vi "Load Device Image.vi"(8 "Error In":errorcluster, 10 "Device Type":u16(ring) items=["chipKIT Uno32", "chipKIT uC32", "chipKIT Max32", "chipKIT DP32"], 11 "Device Family":u16(ring) items=["National Instruments", "Digilent", "Arduino"]) -> (0 "Error Out":errorcluster, 3 "Device Image":picture)   [LabVIEW 2011, in "LVH-LINX.lvlib"]
doc: "Load LINX Device Image"
uses:
  LVH-LINX.lvlib
  <vilib>/LabVIEW Hacker/LVH-Toolbox/Common/LVH-Common.lvlib
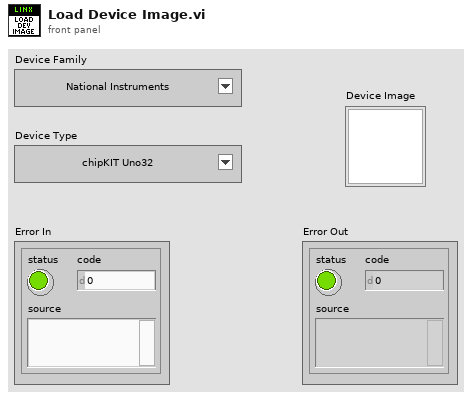
[diagram p1: front panel]
types:
  T1 = typedef "imagedata.ctl" = cluster{"image type":i32, "image depth":i32, "image":u8[], "mask":u8[], "colors":u32[], "Rectangle":cluster{"left":i16, "top":i16, "right":i16, "bottom":i16}}
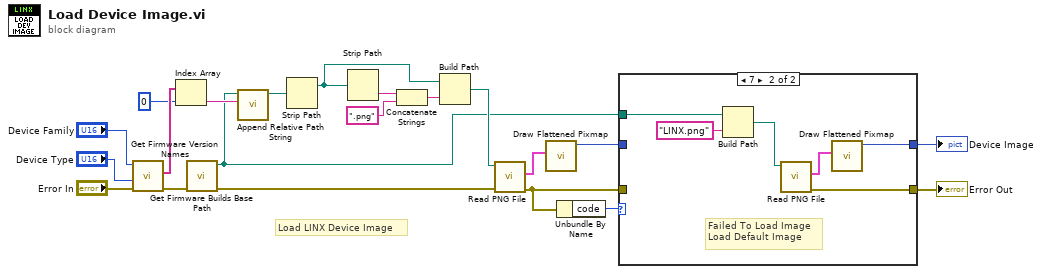
[diagram p0: block diagram]
diagram:
  # "Load LINX Device Image"
  n1 = call "Get Firmware Version Names.vi"("Error In"="Error In", "Device ID"="Device Type", "Device Family"="Device Family") -> ("Error Out"=w20:errorcluster, "Firmware Version Relative Path"=w21:string[])  [unwired: 6 in, 1 out]
  n2 = Index Array(array=w21, index=0) -> (element=w19:string)
  n3 = call "Get Firmware Builds Base Path.vi"("Error In"=w20) -> ("Error Out"=w8:errorcluster, "Firmware Builds Base Path"=w1:path)  [unwired: 9 in]
  n4 = call <vilib>:"Append Relative Path String.vi"("Relative Path"=w19, "Base Path"=w1) -> ("Absolute Path"=w14:path)  [unwired: 9 in]
  n5 = Strip Path(path=w14) -> (stripped path=w11:path)  [unwired: 1 out]
  n6 = Strip Path(path=w11) -> (name=w13:string)  [unwired: 1 out]
  n7 = Concatenate Strings(w13, ".png" ("string")) -> (w10:string)
  n8 = Build Path(base path=w11, name or relative path=w10) -> (appended path=w9:path)
  n9 = call <vilib>:"Read PNG File.vi"("error in (no error)"=w8, "path to PNG file"=w9) -> ("error out"=w5:errorcluster, "image data"=w7:T1)  [unwired: 7 in, 1 out]
  n10 = call <vilib>:"Draw Flattened Pixmap.vi"("image data"=w7) -> ("new picture"=w2:picture)  [unwired: 8 in]
  n11 = Unbundle By Name(w5) -> ("code"=w6:i32)
  n12 = case shown="7" w6 {
    tunnel: w5 -> [w22 _]
    tunnel: [w22 w25] -> w4
    tunnel: [w23 w26] -> w3
    tunnel: w2 -> [w23 _]
    tunnel: w1 -> [_ w29]
    frame 0, Default {
    }
    frame 7 {
      # "Failed To Load Image\nLoad Default Image"
      n13 = Build Path(base path=w29, name or relative path="LINX.png") -> (appended path=w24:path)
      n14 = call <vilib>:"Read PNG File.vi"("path to PNG file"=w24) -> ("error out"=w25:errorcluster, "image data"=w28:T1)  [unwired: 8 in, 1 out]
      n15 = call <vilib>:"Draw Flattened Pixmap.vi"("image data"=w28) -> ("new picture"=w26:picture)  [unwired: 8 in]
    }
  }
  "Error Out" <- w4
  "Device Image" <- w3
